vi "Standard Bus Read--SubVI.vi"(8 "error in":errorcluster, 10 "Register":T1, 11 "Watlow F4T in":refnum<class "Watlow F4T.lvclass">) -> (0 "error out":errorcluster, 1 "Value Out":string, 3 "Watlow F4T out":refnum<class "Watlow F4T.lvclass">)   [LabVIEW 2024, in "Watlow F4T.lvclass"]
uses:
  Watlow F4T.lvclass
  Controls/Standard Bus Register LUT Data--Cluster.ctl
  Watlow F4T.lvclass/Watlow F4T.ctl
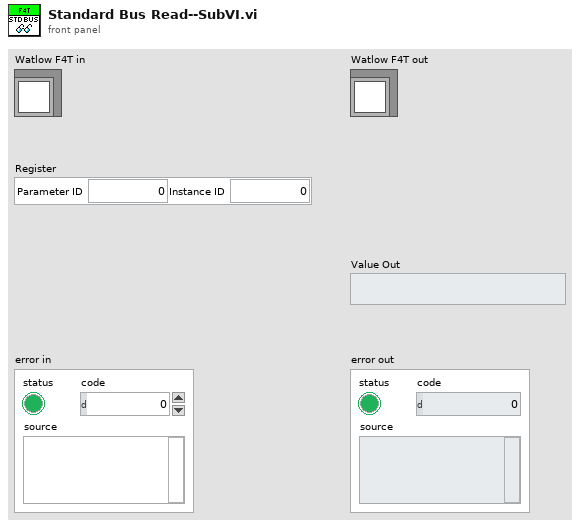
[diagram p1: front panel]
types:
  T1 = typedef "Watlow F4T.lvclass/Standard Bus Register LUT Data--Cluster.ctl" = cluster{"Parameter ID":i32, "Instance ID":i32}
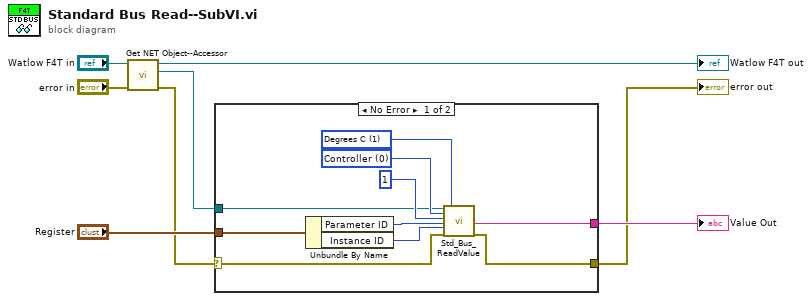
[diagram p0: block diagram]
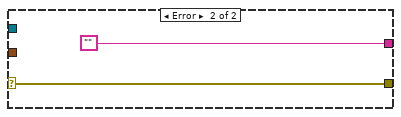
[diagram p2: hidden frame]
diagram:
  n1 = call "Get NET Object--Accessor.vi"("error in (no error)"="error in", "Watlow F4T in"="Watlow F4T in") -> ("error out"=w4:errorcluster, ".NET Object"=w3:refnum<k24>, "Watlow F4T out"=→"Watlow F4T out":refnum<class "Watlow F4T.lvclass">)  [unwired: 7 in]
  n2 = case shown="No Error" w4 {
    selector: w4 -> [w17 w20]
    tunnel: [w15 "" ("Value Out")] -> w7
    tunnel: [w18 w20] -> w1
    tunnel: "Register" -> [w16 _]
    tunnel: w3 -> [w9 _]
    frame No Error {
      w10 = u8 1 items=["Degrees F", "Degrees C"] ("TemperatureUnits")
      w12 = 0 items=["Controller", "RUI", "PC", "CommsCard"] ("DeviceType")
      n3 = Unbundle By Name(w16) -> ("Parameter ID"=w14:i32, "Instance ID"=w13:i32)
      n4 = call <instrlib>:"Std_Bus_ReadValue.vi"("ILabVIEW In"=w9, "DeviceType"=w12, "Zone"=1, "ParameterID"=w14, "InstanceId"=w13, "error in (no error)"=w17, "TemperatureUnits"=w10) -> ("Value Out"=w15:string, "error out"=w18:errorcluster)  [unwired: 10 in, 1 out]
    }
    frame Error {
    }
  }
  "error out" <- w1
  "Value Out" <- w7
